vi "Avancer encodeur.vi"(11 "Distance":dbl) -> (8 "reverse":bool, 9 "Left":bool, 10 "Right":bool)   [LabVIEW 2016]
uses:
  <vilib>/Rock Robotics/WPI/Utilities/WPI_GetSetVariantRefNum.vi
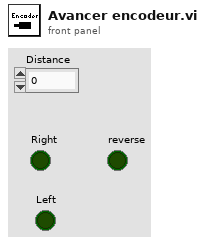
[diagram p1: front panel]
types:
  T1 = typedef "WPI_EncoderDevRef.ctl" = cluster{"DevStatus":errorcluster, "EncoderIndex":T2, "CounterIndex":T3, "DistancePerCount":dbl, "Decoding Type":T4}
  T2 = typedef "FPGA_EncoderIdx.ctl" = enum8{"Enc 0", "Enc 1", "Enc 2", "Enc 3", "Enc 4", "Enc 5", "Enc 6", "Enc 7", "Invalid"}
  T3 = typedef "FPGA_CounterCtrSystemIndex.ctl" = enum8{"Ctr 0", "Ctr 1", "Ctr 2", "Ctr 3", "Ctr 4", "Ctr 5", "Ctr 6", "Ctr 7", "Invalid"}
  T4 = typedef "WPI_EncoderType.ctl" = enum16{"1x", "2x", "4x"}
  T5 = typedef "WPI_RobotDriveDevRef.ctl" = cluster{"DevStatus":errorcluster, "Motors[]":T6[], "Square Inputs":bool, "Max Output":dbl}
  T6 = typedef "WPI_MotorControlDeviceRef.ctl" = cluster{"DeviceStatus":errorcluster, "Type":T7, "PWM":cluster{"PWM Channel":T8, "DeadBand":T9}, "CAN":cluster{"Device Number":u8, "SetOutput VI Ref":variant, "GetOutput VI Ref":variant, "Enable VI Ref":variant, "Disable VI Ref":variant, "Data":variant}, "Invert":bool}
  T7 = typedef "WPI_MotorControlType.ctl" = enum16{"PWM", "CAN"}
  T8 = typedef "FPGA_DIOPWMChannel.ctl" = enum8{"PWM 0", "PWM 1", "PWM 2", "PWM 3", "PWM 4", "PWM 5", "PWM 6", "PWM 7", "PWM 8", "PWM 9", "PWM MXP 0", "PWM MXP 1", "PWM MXP 2", "PWM MXP 3", "PWM MXP 4", "PWM MXP 5", "PWM MXP 6", "PWM MXP 7", "PWM MXP 8", "PWM MXP 9", "Invalid"}
  T9 = typedef "WPI_PWMDeadband.ctl" = cluster{"Name":string, "maxPositivePwm":i32, "minPositivePwm":i32, "centerPwm":i32, "maxNegativePwm":i32, "minNegativePwm":i32, "angularRange":u16}
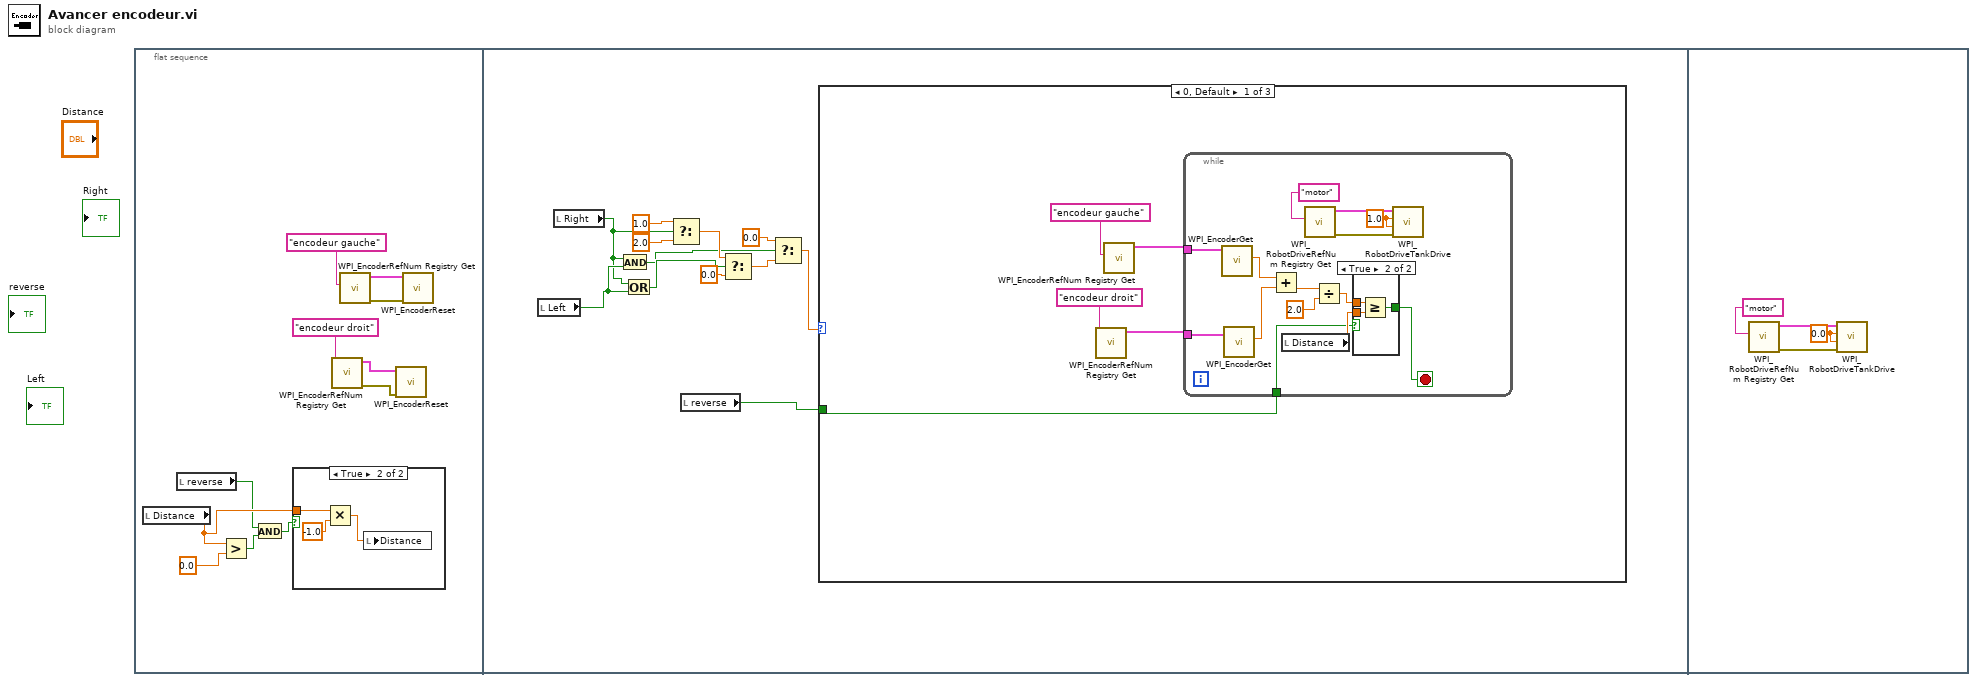
[diagram p0: block diagram]
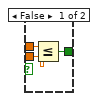
[diagram p3: hidden frame]
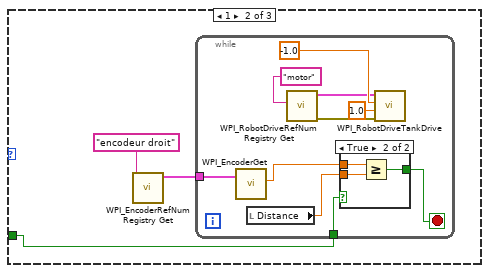
[diagram p4: hidden frame]
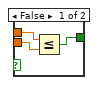
[diagram p5: hidden frame]
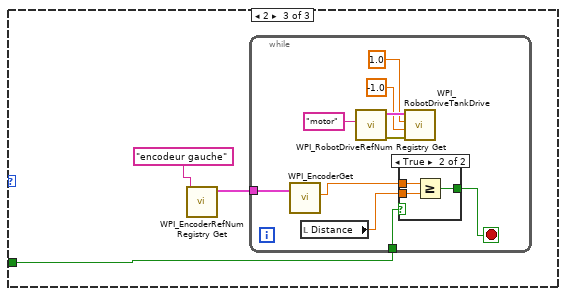
[diagram p6: hidden frame]
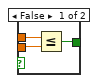
[diagram p7: hidden frame]
diagram:
  n1 = flat-sequence {
    frame #0 {
      n2 = local read "Distance"() -> (w5:dbl)
      n3 = local read "reverse"() -> (w1:bool)
      n4 = Greater?(x=w5, y=0.0) -> (0:w3:bool)
      n5 = And(x=w1, y=w3) -> (x .and. y?=w4:bool)
      n6 = case shown="True" w4 {
        tunnel: w5 -> [_ w14]
        frame False {
        }
        frame True {
          n7 = Multiply(x=w14, y=-1.0) -> (x*y=w12:dbl)
          n8 = local write "Distance"(w12) -> ()
        }
      }
      n9 = call <vilib>:"WPI_EncoderRefNum Registry Get.vi"("refnum name"="encodeur droit") -> ("error out"=w6:errorcluster, "EncoderDevRef"=w7:T1)  [unwired: 9 in]
      n10 = call <vilib>:"WPI_EncoderRefNum Registry Get.vi"("refnum name"="encodeur gauche") -> ("error out"=w8:errorcluster, "EncoderDevRef"=w9:T1)  [unwired: 9 in]
      n11 = call <vilib>:"WPI_EncoderReset.vi"("error in (no error)"=w6, "EncoderDevRef"=w7) -> ()  [unwired: 8 in, 2 out]
      n12 = call <vilib>:"WPI_EncoderReset.vi"("error in (no error)"=w8, "EncoderDevRef"=w9) -> ()  [unwired: 8 in, 2 out]
    }
    frame #1 {
      n13 = local read "Left"() -> (w19:bool)
      n14 = local read "Right"() -> (w18:bool)
      n15 = And(x=w18, y=w19) -> (x .and. y?=w17:bool)
      n16 = Or(x=w18, y=w19) -> (x .or. y?=w20:bool)
      n17 = Select(t=1.0, s=w18, f=2.0) -> (s? t:f=w24:dbl)
      n18 = local read "reverse"() -> (w15:bool)
      n19 = Select(t=w24, s=w20, f=0.0) -> (s? t:f=w21:dbl)
      n20 = Select(t=0.0, s=w17, f=w21) -> (s? t:f=w22:dbl)
      n21 = case shown="0, Default" w22 {
        tunnel: w15 -> [w27 w52 w71]
        frame 0, Default {
          n22 = call <vilib>:"WPI_EncoderRefNum Registry Get.vi"("refnum name"="encodeur droit") -> ("EncoderDevRef"=w30:T1)  [unwired: 9 in, 1 out]
          n23 = call <vilib>:"WPI_EncoderRefNum Registry Get.vi"("refnum name"="encodeur gauche") -> ("EncoderDevRef"=w31:T1)  [unwired: 9 in, 1 out]
          n24 = while {
            tunnel: w30 -> [w45]
            tunnel: w31 -> [w44]
            tunnel: w27 -> [w32]
            stop <- w38 stop-if-true
            w36 = 1.0 ("Left axis value")
            n25 = call <vilib>:"WPI_EncoderGet.vi"("EncoderDevRef"=w44) -> ("Distance"=w43:dbl)  [unwired: 5 in, 5 out]
            n26 = call <vilib>:"WPI_EncoderGet.vi"("EncoderDevRef"=w45) -> ("Distance"=w42:dbl)  [unwired: 5 in, 5 out]
            n27 = Add(x=w43, y=w42) -> (x+y=w41:dbl)
            n28 = local read "Distance"() -> (w37:dbl)
            n29 = call <vilib>:"WPI_RobotDriveRefNum Registry Get.vi"("refnum name"="motor") -> ("error out"=w33:errorcluster, "RobotDriveDevRef"=w34:T5)  [unwired: 9 in]
            n30 = Divide(x=w41, y=2.0) -> (x/y=w39:dbl)
            n31 = case shown="True" w32 {
              tunnel: w39 -> [w48 w51]
              tunnel: [w46 w50] -> w38
              tunnel: w37 -> [w47 w49]
              frame False {
                n32 = Less Or Equal?(x=w48, y=w47) -> (x <= y?=w46:bool)
              }
              frame True {
                n33 = Greater Or Equal?(x=w51, y=w49) -> (x >= y?=w50:bool)
              }
            }
            n34 = call <vilib>:"WPI_RobotDriveTankDrive.vi"("error in (no error)"=w33, "Right axis value"=w36, "Left axis value"=w36, "RobotDriveDevRef"=w34) -> ()  [unwired: 5 in, 3 out]
          }
        }
        frame 1 {
          n35 = call <vilib>:"WPI_EncoderRefNum Registry Get.vi"("refnum name"="encodeur droit") -> ("EncoderDevRef"=w53:T1)  [unwired: 9 in, 1 out]
          n36 = while {
            tunnel: w53 -> [w64]
            tunnel: w52 -> [w55]
            stop <- w63 stop-if-true
            n37 = call <vilib>:"WPI_EncoderGet.vi"("EncoderDevRef"=w64) -> ("Distance"=w62:dbl)  [unwired: 5 in, 5 out]
            n38 = local read "Distance"() -> (w61:dbl)
            n39 = call <vilib>:"WPI_RobotDriveRefNum Registry Get.vi"("refnum name"="motor") -> ("error out"=w58:errorcluster, "RobotDriveDevRef"=w57:T5)  [unwired: 9 in]
            n40 = case shown="True" w55 {
              tunnel: [w65 w70] -> w63
              tunnel: w62 -> [w67 w69]
              tunnel: w61 -> [w66 w68]
              frame False {
                n41 = Less Or Equal?(x=w67, y=w66) -> (x <= y?=w65:bool)
              }
              frame True {
                n42 = Greater Or Equal?(x=w69, y=w68) -> (x >= y?=w70:bool)
              }
            }
            n43 = call <vilib>:"WPI_RobotDriveTankDrive.vi"("error in (no error)"=w58, "Right axis value"=1.0, "Left axis value"=-1.0, "RobotDriveDevRef"=w57) -> ()  [unwired: 5 in, 3 out]
          }
        }
        frame 2 {
          n44 = call <vilib>:"WPI_EncoderRefNum Registry Get.vi"("refnum name"="encodeur gauche") -> ("EncoderDevRef"=w73:T1)  [unwired: 9 in, 1 out]
          n45 = while {
            tunnel: w73 -> [w83]
            tunnel: w71 -> [w74]
            stop <- w82 stop-if-true
            n46 = call <vilib>:"WPI_EncoderGet.vi"("EncoderDevRef"=w83) -> ("Distance"=w81:dbl)  [unwired: 5 in, 5 out]
            n47 = local read "Distance"() -> (w80:dbl)
            n48 = call <vilib>:"WPI_RobotDriveRefNum Registry Get.vi"("refnum name"="motor") -> ("error out"=w77:errorcluster, "RobotDriveDevRef"=w78:T5)  [unwired: 9 in]
            n49 = case shown="True" w74 {
              tunnel: [w84 w89] -> w82
              tunnel: w81 -> [w86 w88]
              tunnel: w80 -> [w85 w87]
              frame False {
                n50 = Less Or Equal?(x=w86, y=w85) -> (x <= y?=w84:bool)
              }
              frame True {
                n51 = Greater Or Equal?(x=w88, y=w87) -> (x >= y?=w89:bool)
              }
            }
            n52 = call <vilib>:"WPI_RobotDriveTankDrive.vi"("error in (no error)"=w77, "Right axis value"=-1.0, "Left axis value"=1.0, "RobotDriveDevRef"=w78) -> ()  [unwired: 5 in, 3 out]
          }
        }
      }
    }
    frame #2 {
      w93 = 0.0 ("Left axis value")
      n53 = call <vilib>:"WPI_RobotDriveRefNum Registry Get.vi"("refnum name"="motor") -> ("error out"=w90:errorcluster, "RobotDriveDevRef"=w91:T5)  [unwired: 9 in]
      n54 = call <vilib>:"WPI_RobotDriveTankDrive.vi"("error in (no error)"=w90, "Right axis value"=w93, "Left axis value"=w93, "RobotDriveDevRef"=w91) -> ()  [unwired: 5 in, 3 out]
    }
  }
